vi "Convert string array to activity log.vi"(4 "Valid DITs Array":bool[](array[boolean]), 5 "Activity Log String Array":string[](array[string])) -> (0 "Activity Log Valid? symbols array":i32[](array[numeric]), 1 "Activity Log Valid? array":bool[](array[boolean]), 2 "Activity Array":T1(array[cluster]))   [LabVIEW 2009]
doc: "Converts the array of activity log to an array of cluster of date string and Activity log string.\n\nAlso formats Activity Log Valid? array and Activity Log Valid? symbols array so that there is 1 boolean and 1 symbol in the array for each element in the Activity array (used to indicate which activities are valid on a line-by-line basis."
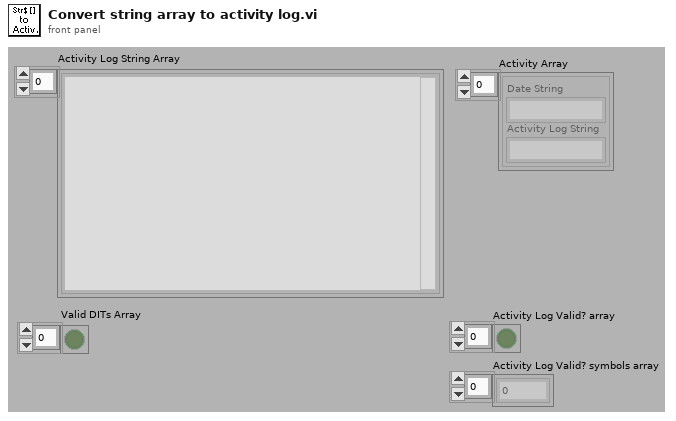
[diagram p1: front panel]
types:
  T1 = cluster{"Date String":string, "Activity Log String":string}[]
  T2 = cluster{"Activity Log String":string, "Activity Log String":string}[]
  T3 = cluster{"Activity Log String":string, "Activity Log String":string}
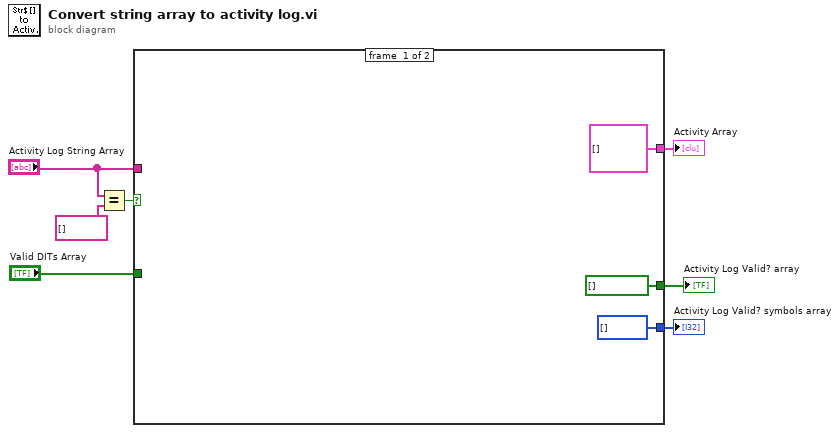
[diagram p0: block diagram]
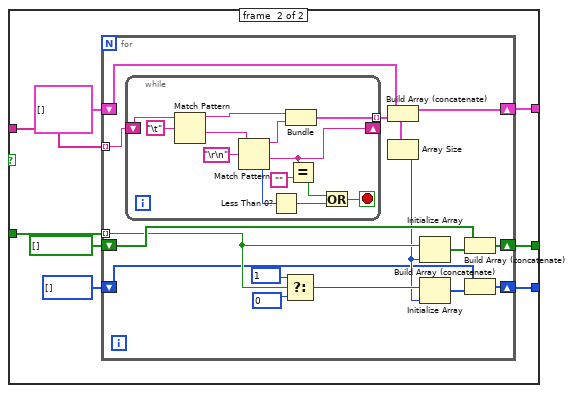
[diagram p2: hidden frame]
diagram:
  n1 = Equal?(x="Activity Log String Array", y=string[] []) -> (x = y?=w5:bool)
  n2 = case shown="False" w5 {
    tunnel: [T2 [] w17] -> w1
    tunnel: "Activity Log String Array" -> [_ w18]
    tunnel: "Valid DITs Array" -> [_ w16]
    tunnel: [bool[] [] w15] -> w3
    tunnel: [i32[] [] w12] -> w2
    frame #0 {
    }
    frame #1 {
      n3 = for {
        tunnel: w18 -> [w33] mode=indexing
        shift-right: [w32] -> w17
        shift-left: T2 [] -> [w30]
        tunnel: w16 -> [w26] mode=indexing
        shift-right: [w29] -> w15
        shift-left: bool[] [] -> [w27]
        shift-right: [w20] -> w12
        shift-left: i32[] [] -> [w19]
        n4 = while {
          tunnel: [w46] -> w31 mode=indexing
          shift-right: [w37] -> _
          shift-left: w33 -> [w42]
          stop <- w35 stop-if-true
          n5 = Match Pattern(string=w42, regular expression="\t") -> (before substring=w39:string, after substring=w40:string)  [unwired: 3 out]
          n6 = Match Pattern(string=w40, regular expression="\r\n") -> (before substring=w43:string, after substring=w37:string, offset past match=w41:i32)  [unwired: 2 out]
          n7 = Less Than 0?(x=w41) -> (x < 0?=w34:bool)
          n8 = Bundle("Activity Log String"=w39, "Activity Log String"=w43) -> (w46:T3)  [unwired: 1 out]
          n9 = Equal?(x=w37, y="") -> (x = y?=w36:bool)
          n10 = Or(x=w36, y=w34) -> (x .or. y?=w35:bool)
        }
        n11 = Select(t=1, s=w26, f=0) -> (s? t:f=w23:i32)
        n12 = Build Array (concatenate)(w30, w31) -> (w32:T2)
        n13 = Array Size(array=w31) -> (size(s)=w22:i32)
        n14 = Initialize Array(w26, w22) -> (w28:bool[])
        n15 = Initialize Array(w23, w22) -> (w21:i32[])
        n16 = Build Array (concatenate)(w27, w28) -> (w29:bool[])
        n17 = Build Array (concatenate)(w19, w21) -> (w20:i32[])
      }
    }
  }
  "Activity Log Valid? array" <- w3
  "Activity Log Valid? symbols array" <- w2
  "Activity Array" <- w1
